vi "GetCommandReturnString.vi"(7 "Timeout (ms)":u32=2000, 8 "Error In":errorcluster, 10 "Command":string, 11 "Sierra M100 In":refnum<visa-resource-name>) -> (0 "Error Out":errorcluster, 1 "Timeout?":bool, 2 "Return String":string, 3 "Sierra M100 Out":refnum<visa-resource-name>)   [LabVIEW 2012, in "Sierra-M100.lvlib"]
uses:
  Sierra-M100.lvlib
  <vilib>/regexp/Match Regular Expression.xnode
panel:
  out "Time Elapsed (ms)":u32
  out "before match":string
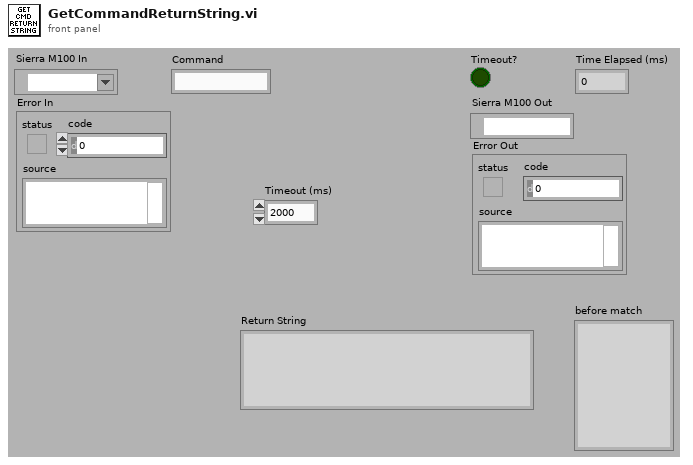
[diagram p1: front panel]
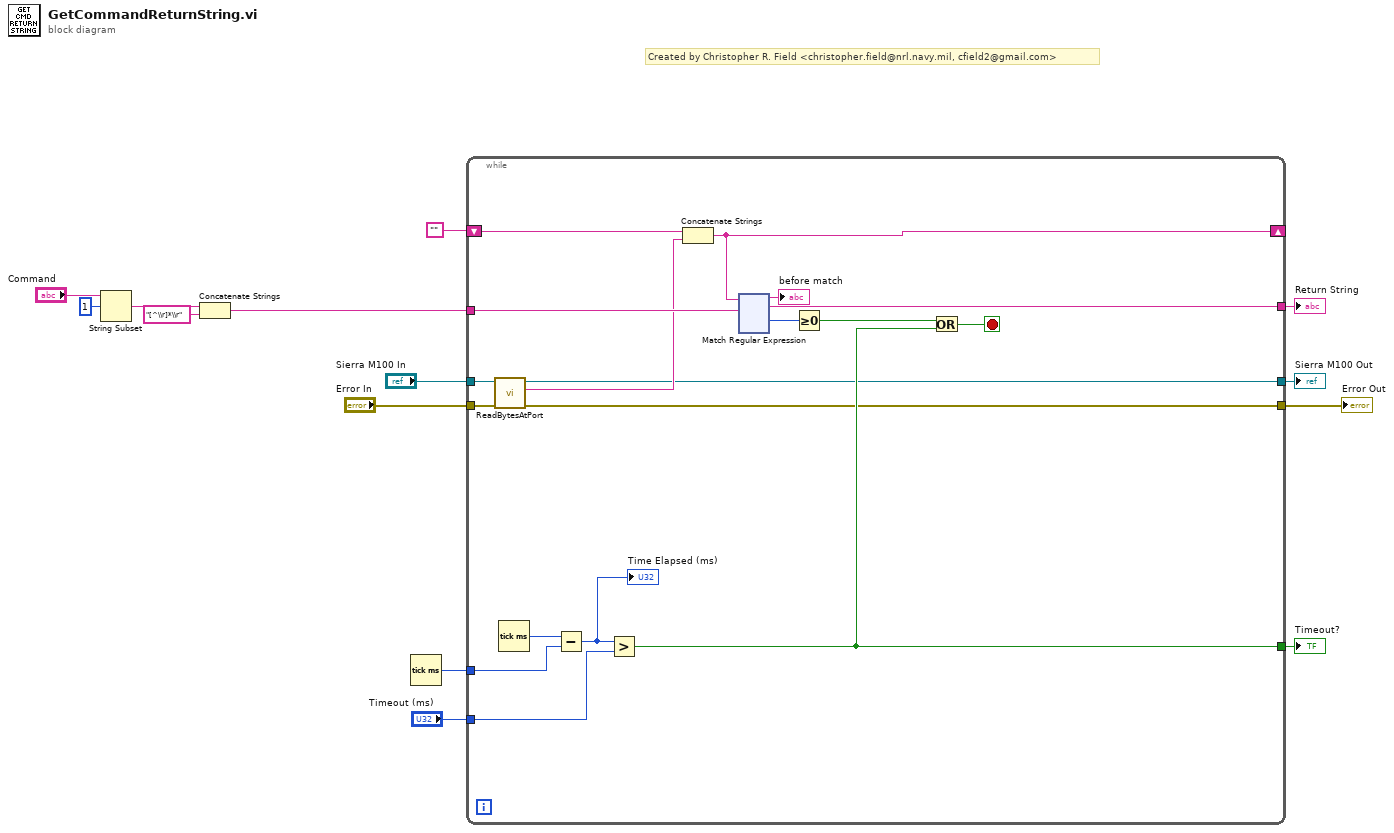
[diagram p0: block diagram]
diagram:
  # "Created by Christopher R. Field <christopher.field@nrl.navy.mil, cfield2@gmail.com>"
  n1 = String Subset(string="Command", offset (0)=1) -> (substring=w7:string)  [unwired: 1 in]
  n2 = Concatenate Strings(w7, "[^\\r]*\\r" ("string")) -> (w5:string)
  n3 = Tick Count (ms)() -> (millisecond timer value=w3:u32)
  n4 = while {
    tunnel: "Sierra M100 In" -> [w16]
    tunnel: "Error In" -> [w15]
    shift-right: [w30] -> _
    shift-left: "" -> [w32]
    tunnel: [w18] -> w11
    tunnel: [w17] -> w10
    tunnel: w5 -> [w31]
    tunnel: [w29] -> w4
    tunnel: w3 -> [w25]
    tunnel: "Timeout (ms)" -> [w23]
    tunnel: [w20] -> w1
    stop <- w21 stop-if-true
    n5 = call "ReadBytesAtPort.vi"("Error In"=w15, "Sierra M100 In"=w16) -> ("Error Out"=w17:errorcluster, "Read Buffer"=w19:string, "Sierra M100 Out"=w18:refnum<visa-resource-name>)  [unwired: 7 in]
    n6 = Tick Count (ms)() -> (millisecond timer value=w26:u32)
    n7 = Subtract(x=w26, y=w25) -> (x-y=w24:u32)
    "Time Elapsed (ms)" <- w24
    n8 = Greater?(x=w24, y=w23) -> (0:w20:bool)
    n9 = Concatenate Strings(w32, w19) -> (w30:string)
    n10 = xnode "Match Regular Expression"("input string"=w30, "regular expression"=w31) -> ("before match"=→"before match":string, "whole match"=w29:string, "offset past match"=w28:i32)  [unwired: 4 in, 2 out]
    n11 = Greater Or Equal To 0?(x=w28) -> (x >= 0?=w22:bool)
    n12 = Or(x=w22, y=w20) -> (x .or. y?=w21:bool)
  }
  "Return String" <- w4
  "Sierra M100 Out" <- w11
  "Error Out" <- w10
  "Timeout?" <- w1
